vi "WFS Example.vi"() -> ()   [LabVIEW 2020]
uses:
  zzz_StateMachineCtrl.ctl
  3D Surface.xctl
  3D Surface Datatype.lvclass
panel:
  in  "Data":enum32{"Wavefront", "Spotfield"}(tab)
  out "3D Surface":refnum<class "3D Plot Datatype.lvclass">[](xcontrol)
  out "Monochrome":u8[][](graph)
  in  "Help":bool
  in  "Tab Control":T1(tab)=enum."Settings"
  in  "Limit to Pupil":i32(ring) caption="Limit to Pupil (No)" items=["Yes"=1, "No"=0]
  in  "Wavefront Type":i32(ring) caption="Wavefront Type (Measured)" items=["Measured", "Reconstructed", "Difference"]
  out "ArrayZernike_um":sgl[](array[numeric])
  out "AZerOrdRms_um":sgl[](array[numeric])
  in  "zernike_orders":i32=3
  out "ArrayDeviationsX":sgl[][](array[numeric])
  out "ArrayDeviationsY":sgl[][](array[numeric])
  out "wf_mean":dbl
  out "wf_min":dbl
  out "wf_weighted_rms":dbl
  out "wf_max":dbl
  out "wf_diff":dbl
  out "wf_rms":dbl
  out "ArrayWavefront":sgl[][](array[numeric])
  out "beam_diameter_x_mm":dbl
  out "beam_centroid_x_mm":dbl
  out "beam_centroid_y_mm":dbl
  out "beam_diameter_y_mm":dbl
  out "ArrayCentroidX":sgl[][](array[numeric])
  out "ArrayCentroidY":sgl[][](array[numeric])
  out "roc_mm":dbl
  in  "Dyn Noise Cut":bool
  in  "Calc Dias":bool
  out "Exposure Time (ms)":dbl caption="Exposure Time Act"
  in  "Resolution Index":i32
  in  "Cancel WF Tilt":i32(ring) caption="Cancel Wavefront Tilt (No)" items=["No", "Yes"]
  in  "ref_idx":i32
  out "spots_x":i32
  out "spots_y":i32
  in  "pupil_dia_x_mm":dbl=2.0
  in  "pupil_center_x_mm":dbl
  in  "pupil_center_y_mm":dbl
  in  "pupil_dia_y_mm":dbl=2.0
  out "Manufacturer":string
  out "InstName":string caption="Instrument Name"
  out "S/N":string
  out "device_id":i32
  in  "error in":errorcluster
  out "error out":errorcluster
  out "user event out":refnum<user-event>
  out "UserEventRefNum":refnum<event-registration>
  in  "State100":T2 caption="States"
  out "State110":bool
  out "Init":bool
  out "Resource Name":string
  in  "Stop":bool
  in  "Measure":bool
  in  "Quit":bool
  # "The documention for the WFS functions can be found in file WFS_Drv.txt."
  # "Calc Beam Centr. Dia"
  # "Calc Spot Centr. Dia Int."
  # "Get Spot Centroids"
  # "Calc Wavefront"
  # "Calc Wavefront Statistics"
  # "Get Spot Deviations"
  # "Zernike Lfs"
  # "Configure Cam"
  # "Set Ref. Plane"
  # "Set Pupil"
  # "Calc Spot to Ref Dev"
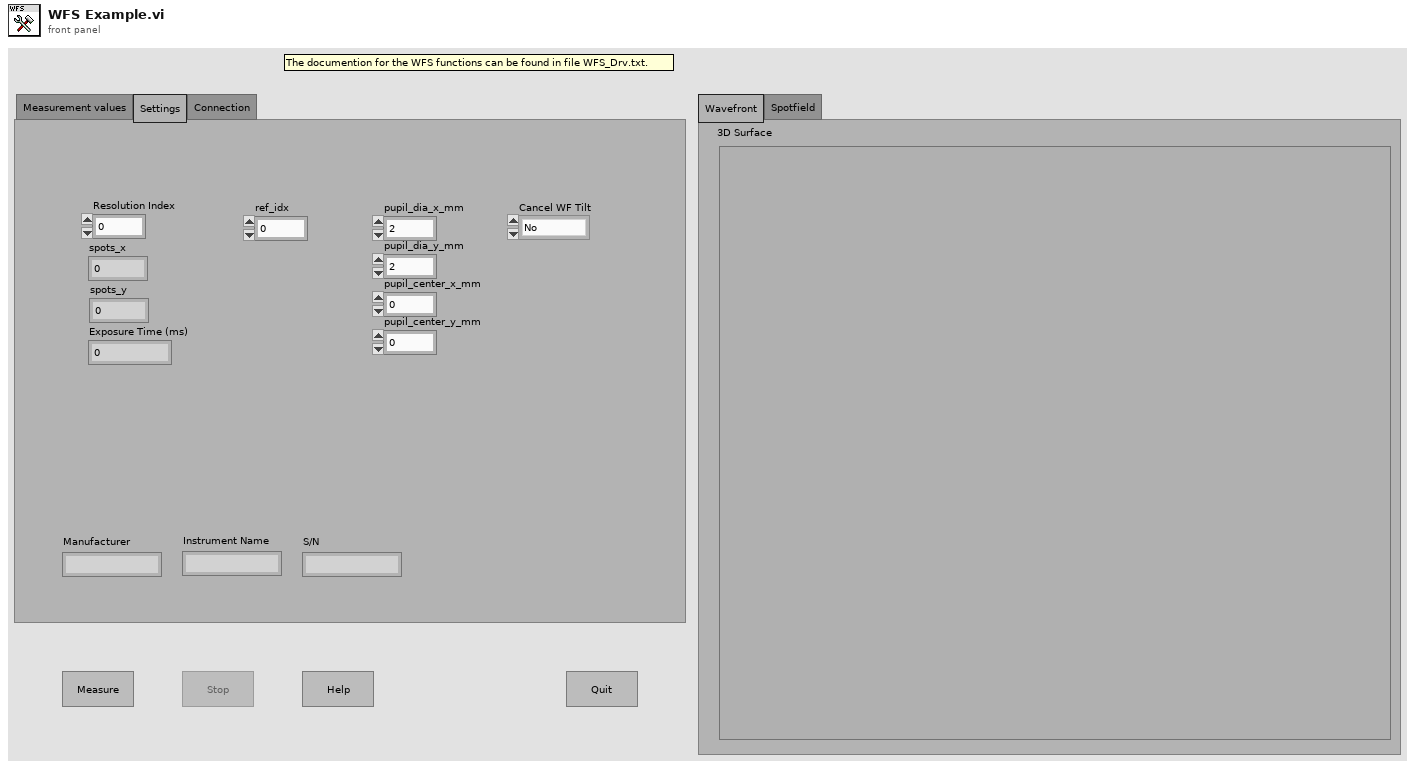
[diagram p1: front panel]
types:
  T1 = enum32{"Measurement values", "Settings", "Connection"}
  T2 = typedef "zzz_StateMachineCtrl.ctl" = enum16{"Initialize", "5", "6", "10", "15", "20", "30", "40", "45", "50", "55", "59", "60", "70", "75", "76", "77", "78", "79", "80", "85", "90", "91", "92", "93", "94", "95", "96", "97", "98", "99", "100", "105", "110", "120", "130", "140", "150", "160", "170", "180", "190", "200", "205", "210", "220", "230", "240", "245", "250", "255", "260", "270", "280", "290", "300", "310", "313", "315", "318", "320", "330", "340", "350", "360", "370", "380", "390", "400", "410", "420", "430", "440", "450", "460", "470", "480", "490", "500", "510", "520", "523", "525", "528", "530", "540", "550", "560", "570", "580", "590", "600", "605", "610", "620", "630", "640", "650", "660", "670", "680", "690", "700", "710", "720", "730", "740", "750", "760", "770", "780", "790", "800", "810", "820", "830", "840", "850", "860", "870", "880", "890", "900", "910", "920", "930", "940", "950", "960", "970", "980", "990", "1000", "1010", "1020", "1030", "1040", "1050", "1060", "1070", "1080", "1090", "1100", "1110", "1120", "1130", "1140", "1150", "1160", "1170", "1180", "1190", "1200", "1210", "1220", "1230", "1240", "1250", "1260", "1270", "1280", "1290", "1300", "Fehler I", "Fehler II", "Fehler III", "Fehler IV", "Fehler V", "Fehler VI", "Fehler VII", "Fehler VIII", "Fehler IX", "Fehler X", "Stop", "Halt Motoren"}
  T3 = enum8{"Enabled", "Disabled", "Disabled and Grayed Out"}
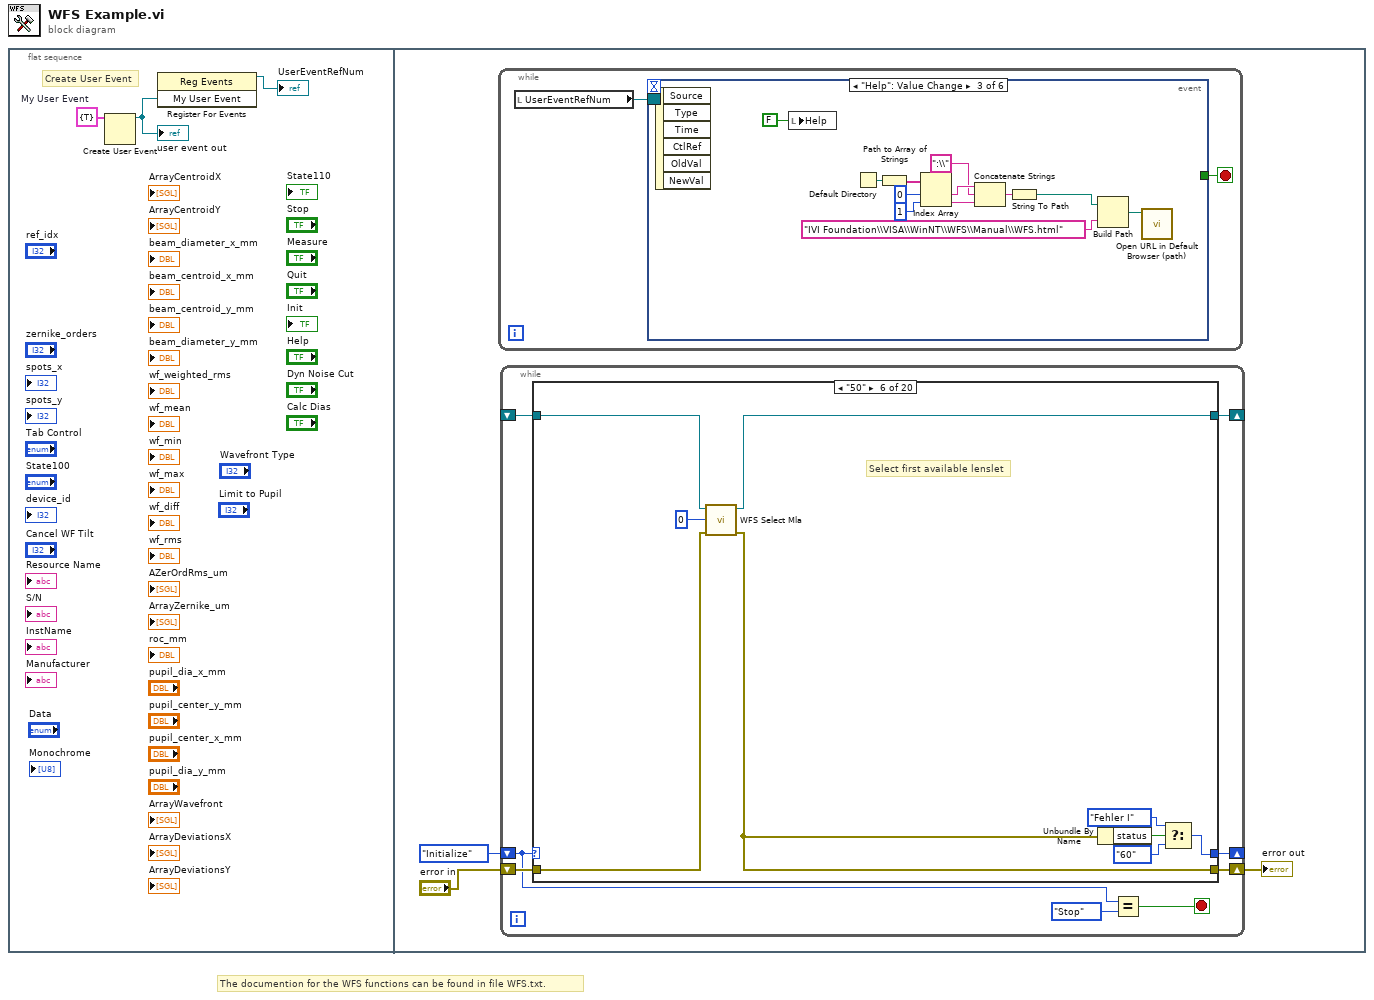
[diagram p0: block diagram]
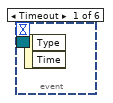
[diagram p2: hidden frame]
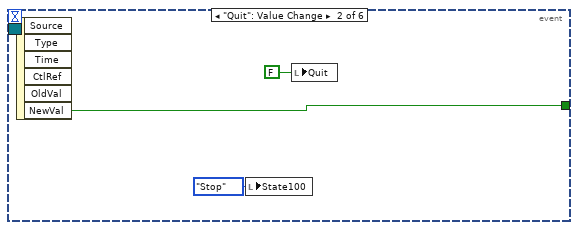
[diagram p3: hidden frame]
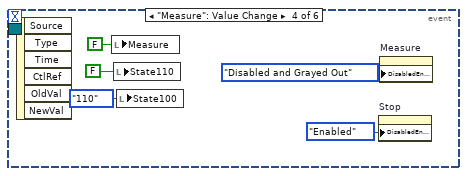
[diagram p4: hidden frame]
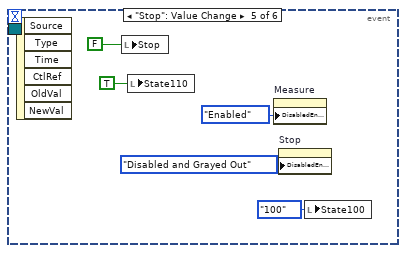
[diagram p5: hidden frame]
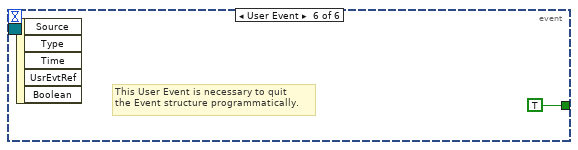
[diagram p6: hidden frame]
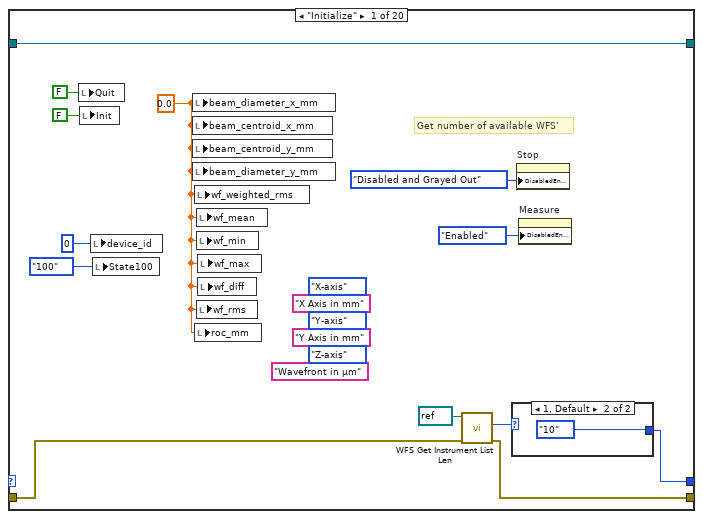
[diagram p7: hidden frame]
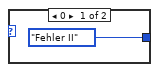
[diagram p8: hidden frame]
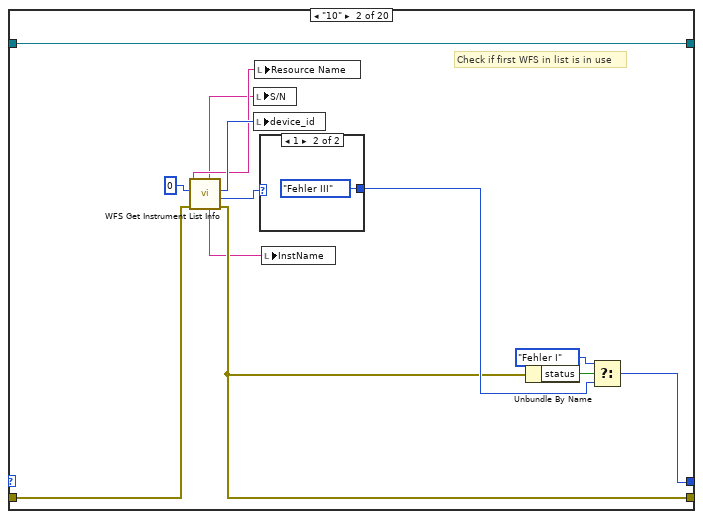
[diagram p9: hidden frame]
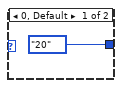
[diagram p10: hidden frame]
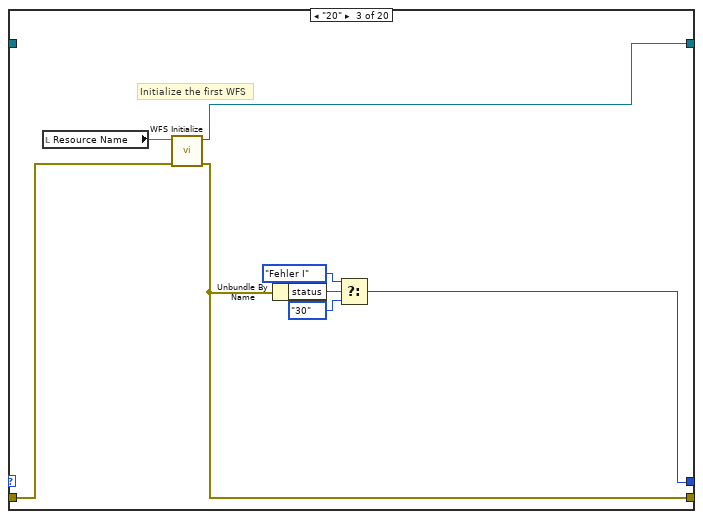
[diagram p11: hidden frame]
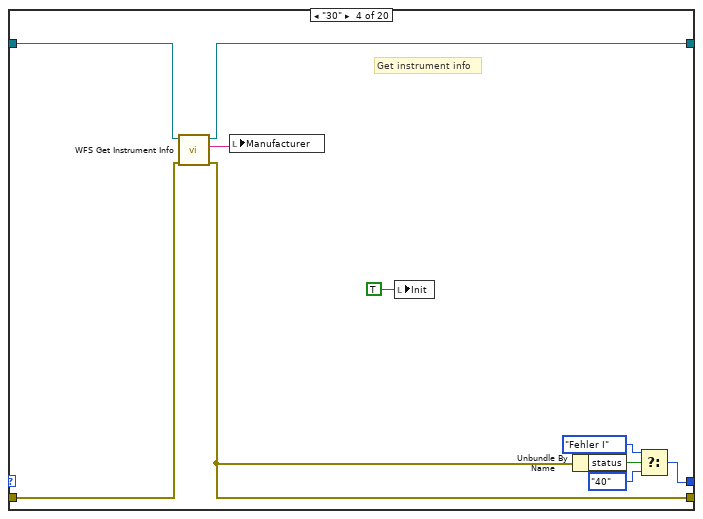
[diagram p12: hidden frame]
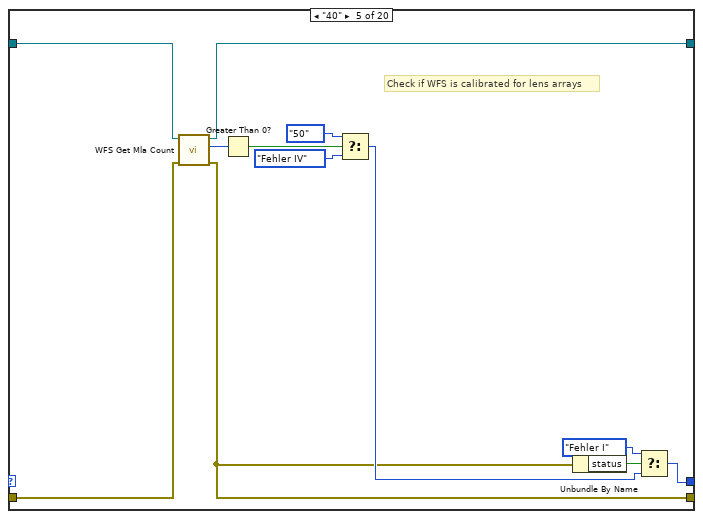
[diagram p13: hidden frame]
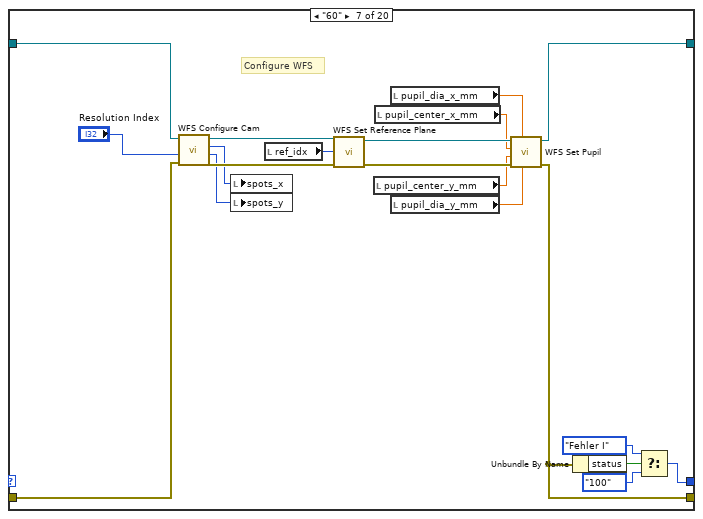
[diagram p14: hidden frame]
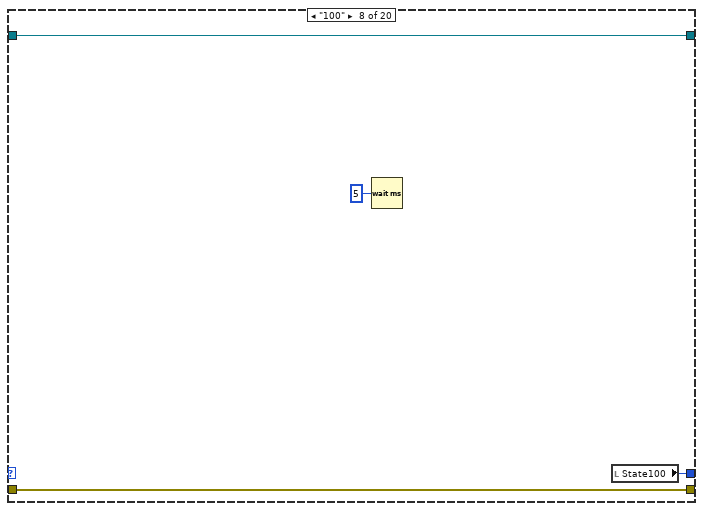
[diagram p15: hidden frame]
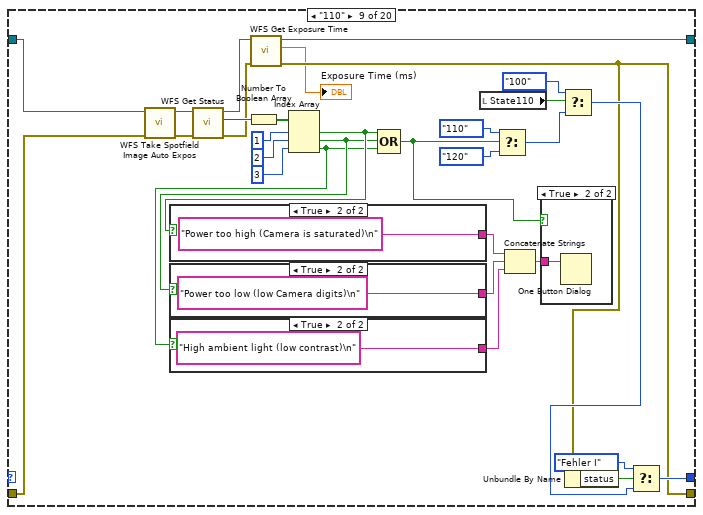
[diagram p16: hidden frame]
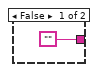
[diagram p18: hidden frame]
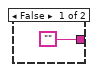
[diagram p19: hidden frame]
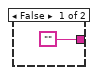
[diagram p20: hidden frame]
diagram:
  # "The documention for the WFS functions can be found in file WFS.txt."
  n1 = flat-sequence {
    frame #0 {
      w3 = cluster{"Boolean":bool} {"Boolean"=TRUE}  # My User Event
      # "Create User Event"
      n2 = Create User Event(user event datatype=w3) -> (user event=w2:refnum<user-event>)  [unwired: 1 in, 1 out]
      "user event out" <- w2
      n3 = register-events(w2) -> (reference out=→"UserEventRefNum":refnum<event-registration>)  [unwired: 2 in, 1 out]
    }
    frame #1 {
      n4 = while {
        stop <- w8 stop-if-true
        n5 = local read "UserEventRefNum"() -> (w7:refnum<event-registration>)
        n6 = event shown="[2] \"Help\": Value Change" {
          selector: w7 -> [_ _ _ _ _ _]
          dyn-events: _ -> [_ _ _ _ _ _]
          timeout: _ -> [_ _ _ _ _ _]
          tunnel: [_ w10 _ _ _ TRUE ("NewVal")] -> w8
          event Timeout {
            n7 = event-data() -> ()  [unwired: 3 out]
          }
          event "Quit": Value Change {
            n8 = event-data() -> ("NewVal"=w10:bool)  [unwired: 6 out]
            n9 = local write "State100"(zzz_StateMachineCtrl."Stop" ("State100")) -> ()
            n10 = local write "Quit"(FALSE ("Quit")) -> ()
          }
          event "Help": Value Change {
            n11 = event-data() -> ()  [unwired: 7 out]
            n12 = local write "Help"(FALSE ("Quit")) -> ()
            n13 = Default Directory() -> (w21:path)
            n14 = Path to Array of Strings(0:w21) -> (2:w20:string[])  [unwired: 1 out]
            n15 = Index Array(array=w20, index #1=0 ("index"), index #2=1 ("index")) -> (element #1=w17:string, element #2=w15:string)
            n16 = Concatenate Strings(w17, ":\\", w15) -> (w16:string)
            n17 = String To Path(string=w16) -> (path=w13:path)
            n18 = Build Path(base path=w13, name or relative path="IVI Foundation\\VISA\\WinNT\\WFS\\Manual\\WFS.html" ("system directory")) -> (appended path=w12:path)
            n19 = call "Open URL in Default Browser (path).vi"("path"=w12) -> ()  [unwired: 5 in, 2 out]
          }
          event "Measure": Value Change {
            n20 = event-data() -> ()  [unwired: 7 out]
            n21 = local write "Measure"(FALSE ("Quit")) -> ()
            n22 = local write "State110"(FALSE ("State110")) -> ()
            n23 = local write "State100"(zzz_StateMachineCtrl."110" ("State100")) -> ()
            n24 = property on="Stop" class="Bool (strict)"("DisabledEnum"=T3."Enabled" ("Disabled")) -> ()  [unwired: 2 in, 2 out]
            n25 = property on="Measure" class="Bool (strict)"("DisabledEnum"=T3."Disabled and Grayed Out" ("Disabled")) -> ()  [unwired: 2 in, 2 out]
          }
          event "Stop": Value Change {
            n26 = event-data() -> ()  [unwired: 7 out]
            n27 = local write "Stop"(FALSE ("Quit")) -> ()
            n28 = local write "State110"(TRUE ("State110")) -> ()
            n29 = property on="Measure" class="Bool (strict)"("DisabledEnum"=T3."Enabled" ("Disabled")) -> ()  [unwired: 2 in, 2 out]
            n30 = property on="Stop" class="Bool (strict)"("DisabledEnum"=T3."Disabled and Grayed Out" ("Disabled")) -> ()  [unwired: 2 in, 2 out]
            n31 = local write "State100"(zzz_StateMachineCtrl."100" ("State100")) -> ()
          }
          event User Event {
            # "This User Event is necessary to quit\nthe Event structure programmatically."
            n32 = event-data() -> ()  [unwired: 6 out]
          }
        }
      }
      n33 = while {
        shift-right: [w42] -> _
        shift-left: zzz_StateMachineCtrl."Initialize" ("States") -> [w37]
        shift-right: [w41] -> _
        shift-left: _ -> [w40]
        shift-right: [w38] -> w4
        shift-left: "error in" -> [w39]
        stop <- w35 stop-if-true
        n34 = case shown="\"50\"" w37 {
          tunnel: [w54 w68 w78 w89 w101 w110 w130 w135 w147 w189 w214 w239 w263 w274 w278 zzz_StateMachineCtrl."Stop" ("States") zzz_StateMachineCtrl."Fehler I" ("States") zzz_StateMachineCtrl."Fehler I" ("States") zzz_StateMachineCtrl."Fehler I" ("States") zzz_StateMachineCtrl."Stop" ("States")] -> w42
          tunnel: [w47 w65 w75 w83 w93 w104 w116 w133 w139 w182 w211 w221 w262 w270 w277 w281 w292 w296 w300 w303] -> w41
          tunnel: w40 -> [w47 w65 _ w85 w94 w107 w117 w133 w143 w179 w213 w229 w248 w271 w277 w281 w292 w296 w300 w303]
          tunnel: w39 -> [w46 w64 w74 w82 w95 w106 w115 w132 w142 w178 w212 w230 w249 w269 w276 w282 w291 w295 w299 w304]
          tunnel: [w45 w63 w73 w81 w91 w103 w114 w132 w137 w187 w210 w215 w261 w268 w276 w282 w291 w295 w299 w304] -> w38
          frame "Initialize" {
            (unwired) "Wavefront in µm" ("Axis:Name Label:Name Label Text")
            (unwired) enum16{"X-axis", "Y-axis", "Z-axis"}."Z-axis" ("Axis:Active Axis")
            (unwired) "Y Axis in mm" ("Axis:Name Label:Name Label Text")
            (unwired) enum16{"X-axis", "Y-axis", "Z-axis"}."Y-axis" ("Axis:Active Axis")
            (unwired) enum16{"X-axis", "Y-axis", "Z-axis"}."X-axis" ("Axis:Active Axis")
            (unwired) "X Axis in mm" ("Axis:Name Label:Name Label Text")
            w49 = 0.0 ("beam_diameter_x_mm")
            # "Get number of available WFS'"
            n35 = local write "Quit"(FALSE ("Quit")) -> ()
            n36 = local write "Init"(FALSE ("Init")) -> ()
            n37 = local write "device_id"(0 ("device_id")) -> ()
            n38 = local write "State100"(zzz_StateMachineCtrl."100" ("State100")) -> ()
            n39 = local write "beam_diameter_x_mm"(w49) -> ()
            n40 = local write "beam_centroid_x_mm"(w49) -> ()
            n41 = local write "beam_centroid_y_mm"(w49) -> ()
            n42 = local write "beam_diameter_y_mm"(w49) -> ()
            n43 = local write "wf_weighted_rms"(w49) -> ()
            n44 = local write "roc_mm"(w49) -> ()
            n45 = local write "wf_mean"(w49) -> ()
            n46 = local write "wf_min"(w49) -> ()
            n47 = local write "wf_rms"(w49) -> ()
            n48 = local write "wf_max"(w49) -> ()
            n49 = local write "wf_diff"(w49) -> ()
            n50 = call "WFS Get Instrument List Len.vi"("error in (no error)"=w46, "instrument handle"=refnum<visa-resource-name> refnum) -> ("error out"=w45:errorcluster, "Instrument Count"=w48:i32)  [unwired: 7 in, 1 out]
            n51 = case shown="1, Default" w48 {
              tunnel: [zzz_StateMachineCtrl."Fehler II" ("States") zzz_StateMachineCtrl."10" ("States")] -> w54
              frame 0 {
              }
              frame 1, Default {
              }
            }
            n52 = property on="Stop" class="Bool (strict)"("DisabledEnum"=T3."Disabled and Grayed Out" ("Disabled")) -> ()  [unwired: 2 in, 2 out]
            n53 = property on="Measure" class="Bool (strict)"("DisabledEnum"=T3."Enabled" ("Disabled")) -> ()  [unwired: 2 in, 2 out]
          }
          frame "10" {
            # "Check if first WFS in list is in use"
            n54 = call "WFS Get Instrument List Info.vi"("error in (no error)"=w64, "Instrument List Index"=0 ("instrument_index")) -> ("error out"=w63:errorcluster, "In Use"=w66:i32, "Device ID"=w62:i32, "Instrument Name"=w58:string, "Instrument SN"=w59:string, "Resource Name"=w60:string)  [unwired: 3 in, 1 out]
            n55 = local write "S/N"(w59) -> ()
            n56 = local write "device_id"(w62) -> ()
            n57 = local write "Resource Name"(w60) -> ()
            n58 = case shown="1" w66 {
              tunnel: [zzz_StateMachineCtrl."20" ("f") zzz_StateMachineCtrl."Fehler III" ("f")] -> w67
              frame 0, Default {
              }
              frame 1 {
              }
            }
            n59 = local write "InstName"(w58) -> ()
            n60 = Unbundle By Name(w63) -> ("status"=w70:bool)
            n61 = Select(t=zzz_StateMachineCtrl."Fehler I" ("States"), s=w70, f=w67) -> (s? t:f=w68:T2)
          }
          frame "20" {
            # "Initialize the first WFS"
            n62 = local read "Resource Name"() -> (w76:string)
            n63 = call "WFS Initialize.vi"("error in (no error)"=w74, "resource name"=w76) -> ("error out"=w73:errorcluster, "instrument handle out"=w75:refnum<visa-resource-name>)  [unwired: 8 in]
            n64 = Unbundle By Name(w73) -> ("status"=w80:bool)
            n65 = Select(t=zzz_StateMachineCtrl."Fehler I" ("States"), s=w80, f=zzz_StateMachineCtrl."30") -> (s? t:f=w78:T2)
          }
          frame "30" {
            # "Get instrument info"
            n66 = call "WFS Get Instrument Info.vi"("error in (no error)"=w82, "instrument handle"=w85) -> ("error out"=w81:errorcluster, "Manufacturer Name"=w84:string, "instrument handle out"=w83:refnum<visa-resource-name>)  [unwired: 4 in, 3 out]
            n67 = local write "Manufacturer"(w84) -> ()
            n68 = local write "Init"(TRUE ("Init")) -> ()
            n69 = Unbundle By Name(w81) -> ("status"=w87:bool)
            n70 = Select(t=zzz_StateMachineCtrl."Fehler I" ("States"), s=w87, f=zzz_StateMachineCtrl."40") -> (s? t:f=w89:T2)
          }
          frame "40" {
            # "Check if WFS is calibrated for lens arrays"
            n71 = call "WFS Get Mla Count.vi"("error in (no error)"=w95, "instrument handle"=w94) -> ("error out"=w91:errorcluster, "MLA Count"=w92:i32, "instrument handle out"=w93:refnum<visa-resource-name>)  [unwired: 7 in]
            n72 = Greater Than 0?(x=w92) -> (x > 0?=w100:bool)
            n73 = Select(t=zzz_StateMachineCtrl."50" ("f"), s=w100, f=zzz_StateMachineCtrl."Fehler IV") -> (s? t:f=w98:T2)
            n74 = Unbundle By Name(w91) -> ("status"=w96:bool)
            n75 = Select(t=zzz_StateMachineCtrl."Fehler I" ("States"), s=w96, f=w98) -> (s? t:f=w101:T2)
          }
          frame "50" {
            # "Select first available lenslet"
            n76 = call "WFS Select Mla.vi"("error in (no error)"=w106, "MLA Index"=0 ("mla_idx"), "instrument handle"=w107) -> ("error out"=w103:errorcluster, "instrument handle out"=w104:refnum<visa-resource-name>)  [unwired: 7 in]
            n77 = Unbundle By Name(w103) -> ("status"=w108:bool)
            n78 = Select(t=zzz_StateMachineCtrl."Fehler I" ("States"), s=w108, f=zzz_StateMachineCtrl."60") -> (s? t:f=w110:T2)
          }
          frame "60" {
            # "Configure WFS"
            n79 = call "WFS Configure Cam.vi"("error in (no error)"=w115, "Cam Resol. Index (1280x1024     640x480       1440x1080         1936x1216          2048x2048)"="Resolution Index", "instrument handle"=w117) -> ("error out"=w126:errorcluster, "Spots Y"=w119:i32, "Spots X"=w118:i32, "instrument handle out"=w127:refnum<visa-resource-name>)  [unwired: 5 in]
            n80 = local write "spots_x"(w118) -> ()
            n81 = local write "spots_y"(w119) -> ()
            n82 = local read "ref_idx"() -> (w113:i32)
            n83 = call "WFS Set Reference Plane.vi"("error in (no error)"=w126, "Reference Index (Internal)"=w113, "instrument handle"=w127) -> ("error out"=w124:errorcluster, "instrument handle out"=w125:refnum<visa-resource-name>)  [unwired: 7 in]
            n84 = local read "pupil_center_y_mm"() -> (w121:dbl)
            n85 = local read "pupil_center_x_mm"() -> (w120:dbl)
            n86 = local read "pupil_dia_x_mm"() -> (w123:dbl)
            n87 = local read "pupil_dia_y_mm"() -> (w122:dbl)
            n88 = call "WFS Set Pupil.vi"("Pupil Diameter Y mm"=w122, "Pupil Diameter X mm"=w123, "error in (no error)"=w124, "Pupil Center Y mm"=w121, "Pupil Center X mm"=w120, "instrument handle"=w125) -> ("error out"=w114:errorcluster, "instrument handle out"=w116:refnum<visa-resource-name>)  [unwired: 4 in]
            n89 = Unbundle By Name(w114) -> ("status"=w128:bool)
            n90 = Select(t=zzz_StateMachineCtrl."Fehler I" ("States"), s=w128, f=zzz_StateMachineCtrl."100") -> (s? t:f=w130:T2)
          }
          frame "100" {
            n91 = Wait (ms)(milliseconds to wait=u32 5) -> ()  [unwired: 1 out]
            n92 = local read "State100"() -> (w135:T2)
          }
          frame "110" {
            n93 = call "WFS Take Spotfield Image Auto Expos.vi"("error in (no error)"=w142, "instrument handle"=w143) -> ("error out"=w144:errorcluster, "instrument handle out"=w145:refnum<visa-resource-name>)  [unwired: 6 in, 2 out]
            n94 = call "WFS Get Status.vi"("error in (no error)"=w144, "instrument handle"=w145) -> ("error out"=w138:errorcluster, "Device Status"=w141:i32, "instrument handle out"=w140:refnum<visa-resource-name>)  [unwired: 7 in]
            n95 = Number To Boolean Array(number=w141) -> (Boolean array=w166:bool[])
            n96 = call "WFS Get Exposure Time.vi"("error in (no error)"=w138, "instrument handle"=w140) -> ("error out"=w137:errorcluster, "Exposure Time Act"=→"Exposure Time (ms)":dbl, "instrument handle out"=w139:refnum<visa-resource-name>)  [unwired: 7 in]
            n97 = Index Array(array=w166, index #1=1 ("index"), index #2=2 ("index"), index #3=3 ("index")) -> (element #1=w160:bool, element #2=w159:bool, element #3=w158:bool)
            n98 = case shown="True" w160 {
              tunnel: ["" "Power too high (Camera is saturated)\n"] -> w157
              frame False {
              }
              frame True {
              }
            }
            n99 = case shown="True" w159 {
              tunnel: ["" "Power too low (low Camera digits)\n"] -> w155
              frame False {
              }
              frame True {
              }
            }
            n100 = case shown="True" w158 {
              tunnel: ["" "High ambient light (low contrast)\n"] -> w156
              frame False {
              }
              frame True {
              }
            }
            n101 = Compound Arithmetic op=OR(w160, w159, w158) -> (w146:bool)
            n102 = local read "State110"() -> (w153:bool)
            n103 = Select(t=zzz_StateMachineCtrl."110" ("States"), s=w146, f=zzz_StateMachineCtrl."120") -> (s? t:f=w152:T2)
            n104 = Concatenate Strings(w157, w155, w156) -> (w154:string)
            n105 = case shown="True" w146 {
              tunnel: w154 -> [_ w167]
              frame False {
              }
              frame True {
                n106 = One Button Dialog(message=w167) -> ()  [unwired: 1 in, 1 out]
              }
            }
            n107 = Select(t=zzz_StateMachineCtrl."100", s=w153, f=w152) -> (s? t:f=w148:T2)
            n108 = Unbundle By Name(w137) -> ("status"=w149:bool)
            n109 = Select(t=zzz_StateMachineCtrl."Fehler I" ("States"), s=w149, f=w148) -> (s? t:f=w147:T2)
          }
          frame "120" {
            n110 = call "WFS Get Spotfield Image Copy.vi"("error in (no error)"=w178, "instrument handle"=w179) -> ("error out"=w176:errorcluster, "Rows"=w175:i32, "ImageBuf"=w180:u8[], "instrument handle out"=w177:refnum<visa-resource-name>, "Columns"=w174:i32)  [unwired: 5 in]
            n111 = Reshape Array(w180, w175, w174) -> (w181:u8[][])
            n112 = local write "Monochrome"(w181) -> ()
            n113 = call "WFS Calc Beam Centroid Dia.vi"("error in (no error)"=w176, "instrument handle"=w177) -> ("error out"=w187:errorcluster, "Beam Centroid Y mm"=w184:dbl, "Beam Centroid X mm"=w185:dbl, "instrument handle out"=w182:refnum<visa-resource-name>, "Beam Diameter X mm"=w183:dbl, "Beam Diameter Y mm"=w186:dbl)  [unwired: 4 in]
            n114 = local write "beam_diameter_x_mm"(w183) -> ()
            n115 = local write "beam_diameter_y_mm"(w186) -> ()
            n116 = local write "beam_centroid_x_mm"(w185) -> ()
            n117 = local write "beam_centroid_y_mm"(w184) -> ()
            n118 = Unbundle By Name(w187) -> ("status"=w190:bool)
            n119 = Select(t=zzz_StateMachineCtrl."Fehler I" ("States"), s=w190, f=zzz_StateMachineCtrl."130") -> (s? t:f=w189:T2)
          }
          frame "130" {
            n120 = local read "Dyn Noise Cut"() -> (w202:bool)
            n121 = local read "Calc Dias"() -> (w201:bool)
            n122 = call "WFS Calc Spots Centr Dia Intens.vi"("error in (no error)"=w212, "Calculate Diameters (Off)"=w201, "Dynamic Noise Cut (On)"=w202, "instrument handle"=w213) -> ("error out"=w207:errorcluster, "instrument handle out"=w206:refnum<visa-resource-name>)  [unwired: 6 in]
            n123 = call "WFS Get Spot Centroids.vi"("error in (no error)"=w207, "instrument handle"=w206) -> ("error out"=w205:errorcluster, "Array Centroid Y"=w197:sgl[], "Array Centroid X"=w199:sgl[], "instrument handle out"=w203:refnum<visa-resource-name>)  [unwired: 6 in]
            n124 = Reshape Array(w199, 80 ("dimension size"), 80 ("dimension size")) -> (w198:sgl[][])
            n125 = Reshape Array(w197, 80 ("dimension size"), 80 ("dimension size")) -> (w196:sgl[][])
            n126 = local write "ArrayCentroidY"(w196) -> ()
            n127 = local read "Cancel WF Tilt"() -> (w200:i32)
            n128 = local write "ArrayCentroidX"(w198) -> ()
            n129 = call "WFS Calc Spot To Reference Deviations.vi"("error in (no error)"=w205, "Cancel Wavefront Tilt (No)"=w200, "instrument handle"=w203) -> ("error out"=w210:errorcluster, "instrument handle out"=w211:refnum<visa-resource-name>)  [unwired: 7 in]
            n130 = Unbundle By Name(w210) -> ("status"=w204:bool)
            n131 = Select(t=zzz_StateMachineCtrl."Fehler I" ("States"), s=w204, f=zzz_StateMachineCtrl."140") -> (s? t:f=w214:T2)
          }
          frame "140" {
            w233 = 0 ("index")
            n132 = local read "Wavefront Type"() -> (w235:i32)
            n133 = local read "Limit to Pupil"() -> (w236:i32)
            n134 = call "WFS Calc Wavefront.vi"("error in (no error)"=w230, "Limit to Pupil (No)"=w236, "Wavefront Type (Measured)"=w235, "instrument handle"=w229) -> ("error out"=w232:errorcluster, "Array Wavefront"=w226:sgl[], "instrument handle out"=w231:refnum<visa-resource-name>)  [unwired: 5 in]
            n135 = local read "spots_y"() -> (w223:i32)
            n136 = local read "spots_x"() -> (w222:i32)
            n137 = Reshape Array(w226, 80 ("dimension size"), 80 ("dimension size")) -> (w225:sgl[][])
            n138 = local write "ArrayWavefront"(w225) -> ()
            n139 = Array Subset(array=w225, index (row)=w233, length (row)=w223, index (col)=w233, length (col)=w222) -> (w224:sgl[][])
            n140 = Transpose 2D Array(2D array=w224) -> (transposed array=w219:sgl[][])
            n141 = call "WFS Get XY Scale.vi"("error in (no error)"=w232, "instrument handle"=w231) -> ("error out"=w216:errorcluster, "Array Scale Y"=w217:sgl[], "Array Scale X"=w218:sgl[], "instrument handle out"=w221:refnum<visa-resource-name>)  [unwired: 6 in]
            n142 = call "Plot Helper (Vector).vi"("z matrix"=w219, "error in (no error)"=w216, "y vector"=w217, "x vector"=w218) -> ("error out"=w215:errorcluster, "3D Plot lvclass Array out"=→"3D Surface":refnum<class "3D Plot Datatype.lvclass">[])  [unwired: 6 in]
            n143 = Unbundle By Name(w215) -> ("status"=w234:bool)
            n144 = Select(t=zzz_StateMachineCtrl."Fehler I" ("States"), s=w234, f=zzz_StateMachineCtrl."150") -> (s? t:f=w239:T2)
          }
          frame "150" {
            n145 = call "WFS Calc Wavefront Statistics.vi"("error in (no error)"=w249, "instrument handle"=w248) -> ("error out"=w252:errorcluster, "Max"=w253:dbl, "Min"=w254:dbl, "instrument handle out"=w257:refnum<visa-resource-name>, "Diff"=w251:dbl, "Mean"=w255:dbl, "RMS"=w250:dbl, "Weighted RMS"=w256:dbl)  [unwired: 2 in]
            n146 = local write "wf_weighted_rms"(w256) -> ()
            n147 = local write "wf_mean"(w255) -> ()
            n148 = local write "wf_min"(w254) -> ()
            n149 = local write "wf_max"(w253) -> ()
            n150 = local write "wf_diff"(w251) -> ()
            n151 = local write "wf_rms"(w250) -> ()
            n152 = call "WFS Get Spot Deviations.vi"("error in (no error)"=w252, "instrument handle"=w257) -> ("error out"=w261:errorcluster, "Array Deviations Y"=w241:sgl[], "Array Deviations X"=w242:sgl[], "instrument handle out"=w262:refnum<visa-resource-name>)  [unwired: 6 in]
            n153 = Reshape Array(w242, 80 ("dimension size"), 80 ("dimension size")) -> (w243:sgl[][])
            n154 = Reshape Array(w241, 80 ("dimension size"), 80 ("dimension size")) -> (w240:sgl[][])
            n155 = local write "ArrayDeviationsX"(w243) -> ()
            n156 = local write "ArrayDeviationsY"(w240) -> ()
            n157 = Unbundle By Name(w261) -> ("status"=w258:bool)
            n158 = Select(t=zzz_StateMachineCtrl."Fehler I" ("States"), s=w258, f=zzz_StateMachineCtrl."160") -> (s? t:f=w263:T2)
          }
          frame "160" {
            n159 = local read "zernike_orders"() -> (w264:i32)
            n160 = call "WFS Zernike Lsf.vi"("error in (no error)"=w269, "Zernike Orders"=w264, "instrument handle"=w271) -> ("error out"=w268:errorcluster, "Array Zernike um"=w266:sgl[], "instrument handle out"=w270:refnum<visa-resource-name>, "Array Zernike Orders um"=w265:sgl[], "RoC mm"=w267:dbl)  [unwired: 4 in]
            n161 = local write "roc_mm"(w267) -> ()
            n162 = local write "ArrayZernike_um"(w266) -> ()
            n163 = local write "AZerOrdRms_um"(w265) -> ()
            n164 = Unbundle By Name(w268) -> ("status"=w272:bool)
            n165 = Select(t=zzz_StateMachineCtrl."Fehler I" ("States"), s=w272, f=zzz_StateMachineCtrl."170") -> (s? t:f=w274:T2)
          }
          frame "170" {
            w278 = zzz_StateMachineCtrl."100" ("State100")
            n166 = property on="Measure" class="Bool (strict)"("DisabledEnum"=T3."Enabled" ("Disabled")) -> ()  [unwired: 2 in, 2 out]
            n167 = property on="Stop" class="Bool (strict)"("DisabledEnum"=T3."Disabled and Grayed Out" ("Disabled")) -> ()  [unwired: 2 in, 2 out]
            n168 = local write "State100"(w278) -> ()
          }
          frame "Fehler I" {
            # "Fire User Event"
            n169 = local read "user event out"() -> (w287:refnum<user-event>)
            n170 = Unbundle By Name(w282) -> ("status"=w284:bool, "code"=w283:i32)
            n171 = Generate User Event(user event=w287, event data cluster=cluster{"Boolean":bool} {"Boolean"=TRUE} ("event data")) -> ()  [unwired: 2 in, 2 out]
            n172 = case shown="True" w284 {
              tunnel: w283 -> [_ w290]
              tunnel: w281 -> [_ w288]
              frame False {
              }
              frame True {
                n173 = call "WFS Error Message.vi"("Error Code"=w290, "instrument handle"=w288) -> ("Error Message"=w289:string)  [unwired: 7 in, 2 out]
                n174 = One Button Dialog(message=w289) -> ()  [unwired: 1 in, 1 out]
              }
            }
          }
          frame "Fehler II" {
            n175 = One Button Dialog(message="No device found!") -> ()  [unwired: 1 in, 1 out]
          }
          frame "Fehler III" {
            n176 = One Button Dialog(message="Selected device is in use by another application!") -> ()  [unwired: 1 in, 1 out]
          }
          frame "Fehler IV" {
            n177 = One Button Dialog(message="The WFS is not calibrated.") -> ()  [unwired: 1 in, 1 out]
          }
          frame "Stop", Default {
            n178 = local read "Init"() -> (w305:bool)
            n179 = case shown="True" w305 {
              tunnel: w303 -> [_ w307]
              frame False {
              }
              frame True {
                n180 = call "WFS Close.vi"("instrument handle"=w307) -> ()  [unwired: 10 in, 1 out]
                n181 = local write "Init"(FALSE ("Init")) -> ()
              }
            }
          }
        }
        n182 = Equal?(x=w37, y=zzz_StateMachineCtrl."Stop") -> (x = y?=w35:bool)
      }
      "error out" <- w4
    }
  }
